vi "SetCompensationTemperature.vi"(8 "error in":errorcluster, 9 "Temperature":sgl, 10 "Address":u8, 11 "VISA resource name":refnum<visa-resource-name>) -> (0 "error out":errorcluster, 1 "Raw Response":string, 2 "SetTemp":dbl, 3 "VISA resource name out":refnum<visa-resource-name>)   [LabVIEW 2020, in "driver_flodx_ph_probe.lvlib"]
doc: "Sets the compensation temperature of the ph probe"
uses:
  <instrlib>/RxnRover/FloDx Ph Probe Driver/driver_flodx_ph_probe.lvlib
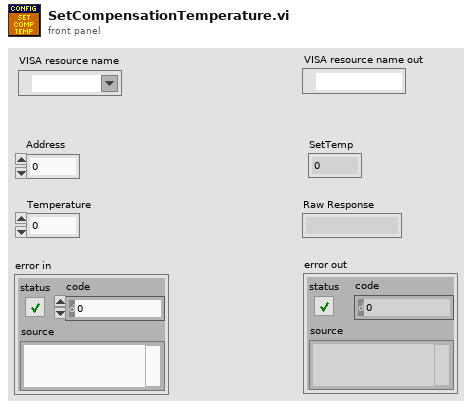
[diagram p1: front panel]
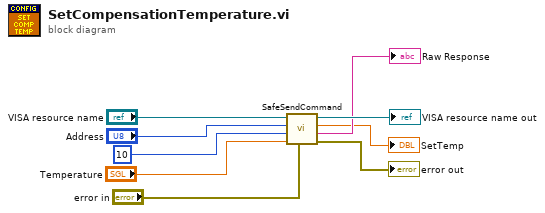
[diagram p0: block diagram]
diagram:
  n1 = call <instrlib>:"SafeSendCommand.vi"("error in"="error in", "Parameter"="Temperature", "Command #"=u8 10 ("Command"), "Address #"="Address", "VISA resource name"="VISA resource name") -> ("error out"=→"error out":errorcluster, "Raw Response"=→"Raw Response":string, "Value"=→"SetTemp":dbl, "VISA resource name out"=→"VISA resource name out":refnum<visa-resource-name>)  [unwired: 3 in]
